vi "GetIntegrationTime.vi"(8 "error in":errorcluster {"code" format="%.0x"}, 10 "ArgIndex(0)":i32, 11 "Args":string[](array[string])) -> (0 "error out":errorcluster {"code" format="%.0x"}, 2 "ExposureTime(mSec)":string, 3 "ExposureTime(mSec)":dbl)   [LabVIEW 2020]
doc: "Retreive the exposure time from the 'Args' array"
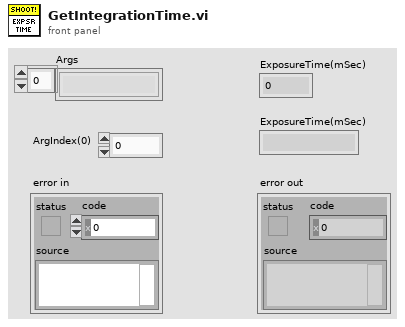
[diagram p1: front panel]
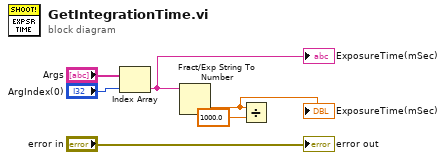
[diagram p0: block diagram]
diagram:
  n1 = Index Array(array="Args", index="ArgIndex(0)") -> (element=w4:string)
  "ExposureTime(mSec)" <- w4
  n2 = Fract/Exp String To Number(string=w4) -> (number=w1:dbl)  [unwired: 3 in, 1 out]
  "ExposureTime(mSec)" <- w1
  n3 = Divide(x=w1, y=1000.0) -> ()  [unwired: 1 out]
  "error out" <- "error in"
